vi "Calculate Response Internal.vi"(10 "Inputs":dbl[](array[numeric]), 11 "Neural Network In":T1={"Weigths"=[], "Last Layer Linear"=TRUE, "Add Bias Inputs"=TRUE, "# Inputs"=0, "# Output Neurons/Outputs"=0, "Inputs Scaling"={"X Scaling Vector"=[], "Y Scaling Vector"=[]}, "Outputs Scaling"={"X Scaling Vector"=[], "Y Scaling Vector"=[]}}) -> (0 "All Inputs":T4[](array[typedef]), 1 "Derrivatives":T4[](array[typedef]), 2 "Outputs":dbl[](array[numeric]), 3 "Neural Network Out":T1={"Weigths"=[], "Last Layer Linear"=TRUE, "Add Bias Inputs"=TRUE, "# Inputs"=0, "# Output Neurons/Outputs"=0, "Inputs Scaling"={"X Scaling Vector"=[], "Y Scaling Vector"=[]}, "Outputs Scaling"={"X Scaling Vector"=[], "Y Scaling Vector"=[]}})   [LabVIEW 2011, in "Super Simple Neural Network.lvlib"]
uses:
  Super Simple Neural Network.lvlib
  <vilib>/Analysis/NI_AALBase.lvlib
  <vilib>/Analysis/baseanly.llb/A x Vector.vi
  Types/1D Array.ctl
  Types/2D Array.ctl
  Types/Neural Network.ctl
  Types/Scaling Info.ctl
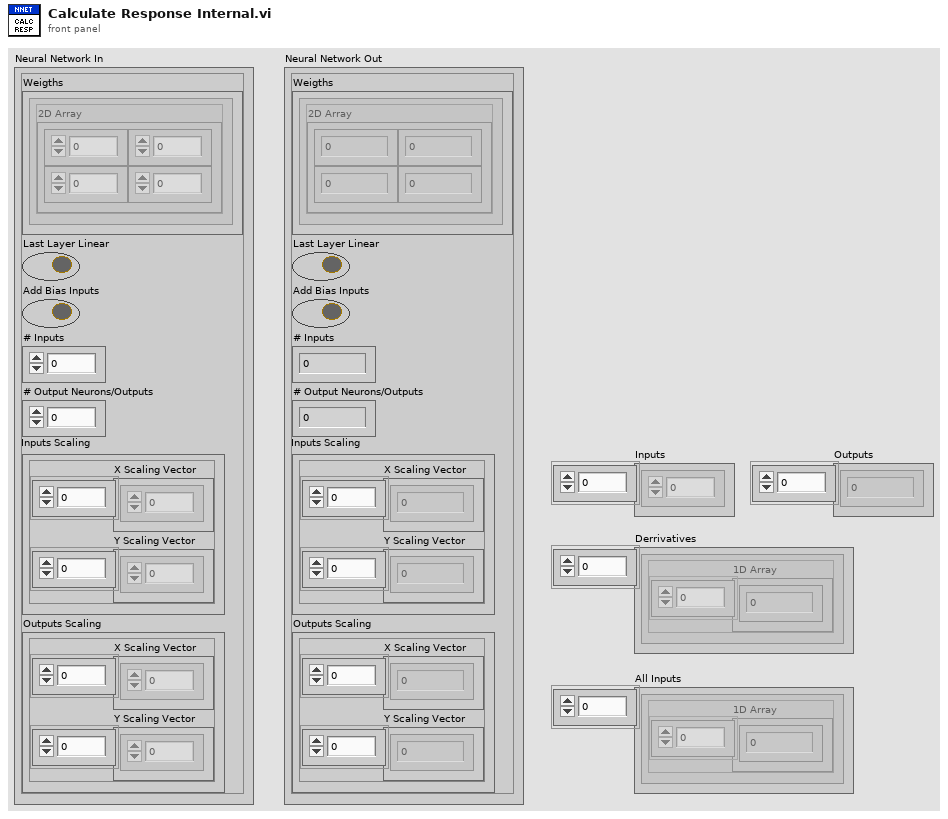
[diagram p1: front panel]
types:
  T1 = typedef "Super Simple Neural Network.lvlib/Neural Network.ctl" = cluster{"Weigths":T2[], "Last Layer Linear":bool, "Add Bias Inputs":bool, "# Inputs":u32, "# Output Neurons/Outputs":u32, "Inputs Scaling":T3, "Outputs Scaling":T3}
  T2 = typedef "Super Simple Neural Network.lvlib/2D Array.ctl" = cluster{"2D Array":dbl[][]}
  T3 = typedef "Super Simple Neural Network.lvlib/Scaling Info.ctl" = cluster{"X Scaling Vector":dbl[], "Y Scaling Vector":dbl[]}
  T4 = typedef "Super Simple Neural Network.lvlib/1D Array.ctl" = cluster{"1D Array":dbl[]}
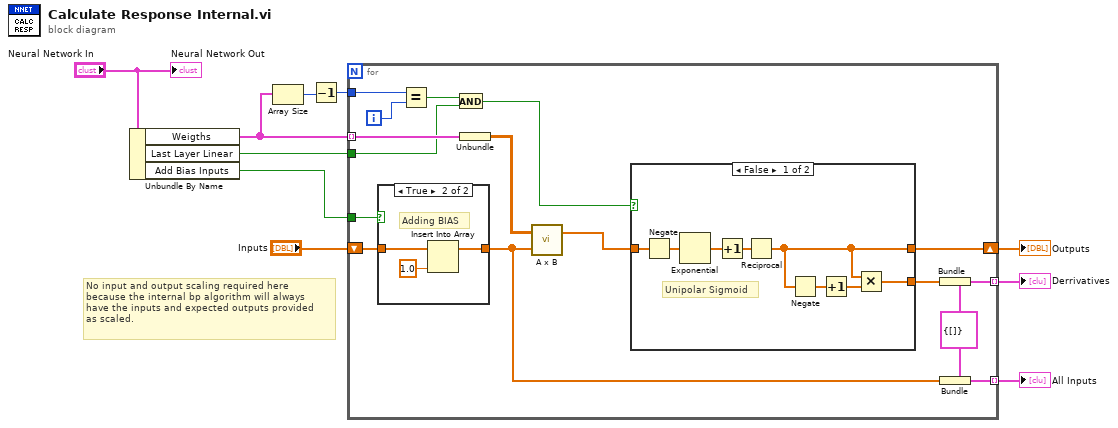
[diagram p0: block diagram]
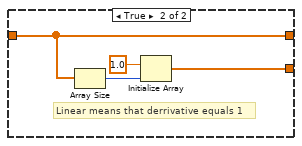
[diagram p3: hidden frame]
diagram:
  # "No input and output scaling required here\nbecause the internal bp algorithm will always \nhave the inputs and expected outputs provided\nas scaled."
  n1 = Unbundle By Name("Neural Network In") -> ("Weigths"=w2:T2[], "Last Layer Linear"=w1:bool, "Add Bias Inputs"=w3:bool)
  n2 = Array Size(array=w2) -> (size(s)=w5:i32)
  n3 = Decrement(x=w5) -> (x-1=w4:i32)
  n4 = for {
    shift-right: [w20] -> w8
    shift-left: "Inputs" -> [w19]
    tunnel: [w24] -> w7 mode=indexing
    tunnel: w2 -> [w26] mode=indexing
    tunnel: [w23] -> w6 mode=indexing
    tunnel: w4 -> [w16]
    tunnel: w3 -> [w14]
    tunnel: w1 -> [w11]
    i -> [w13]
    w22 = T4 {"1D Array"=[]} ("1D Array")
    n5 = case shown="True" w14 {
      tunnel: w19 -> [w27 w29]
      tunnel: [w27 w28] -> w18
      frame False {
      }
      frame True {
        # "Adding BIAS"
        n6 = Insert Into Array(array=w29, new element=1.0 ("new element/subarray")) -> (w28:dbl[])  [unwired: 1 in]
      }
    }
    n7 = Equal?(x=w16, y=w13) -> (x = y?=w15:bool)
    n8 = And(x=w15, y=w11) -> (x .and. y?=w12:bool)
    n9 = Unbundle(w26) -> ("2D Array"=w25:dbl[][])
    n10 = call-poly <vilib>:"A x B.vi"("Vector"=w18, "A"=w25) -> ("A x Vector"=w17:dbl[])  [unwired: 1 out]
    n11 = case shown="False" w12 {
      tunnel: [w33 w40] -> w21
      tunnel: [w32 w42] -> w20
      tunnel: w17 -> [w31 w42]
      frame False {
        # "Unipolar Sigmoid"
        n12 = Negate(x=w31) -> (-x=w38:dbl[])
        n13 = Exponential(1:w38) -> (0:w37:dbl[])
        n14 = Increment(x=w37) -> (x+1=w36:dbl[])
        n15 = Reciprocal(x=w36) -> (1/x=w32:dbl[])
        n16 = Negate(x=w32) -> (-x=w35:dbl[])
        n17 = Increment(x=w35) -> (x+1=w34:dbl[])
        n18 = Multiply(x=w32, y=w34) -> (x*y=w33:dbl[])
      }
      frame True {
        # "Linear means that derrivative equals 1"
        n19 = Array Size(array=w42) -> (size(s)=w41:i32)
        n20 = Initialize Array(1.0 ("new element/subarray"), w41) -> (w40:dbl[])
      }
    }
    n21 = Bundle(cluster=w22, "1D Array"=w21) -> (w24:T4)
    n22 = Bundle(cluster=w22, "1D Array"=w18) -> (w23:T4)
  }
  "Outputs" <- w8
  "Derrivatives" <- w7
  "All Inputs" <- w6
  "Neural Network Out" <- "Neural Network In"
